vi "Arm Logic.vi"(8 "Button":bool=TRUE, 10 "Claw":bool=TRUE, 11 "Tote Count":dbl format="%#_13g") -> ()   [LabVIEW 2014]
uses:
  TypeDefs/SRE Enum.ctl
  Support Code/Robot Global Data.vi
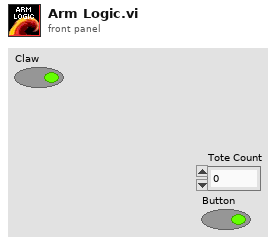
[diagram p1: front panel]
types:
  T1 = typedef "SRE Enum.ctl" = enum16{"Start", "Run", "End"}
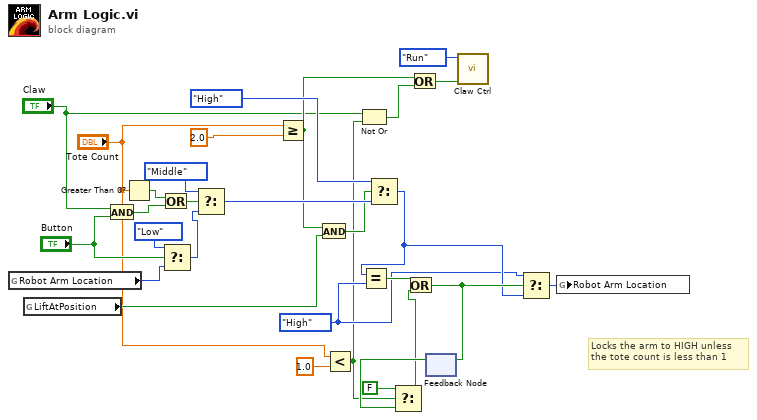
[diagram p0: block diagram]
diagram:
  w12 = enum16{"High", "Middle", "Low"}."High" ("y")
  # "Locks the arm to HIGH unless\nthe tote count is less than 1"
  n1 = global read "Robot Global Data.vi" "Robot Arm Location"() -> (w6:enum16{"High", "Middle", "Low"})
  n2 = global read "Robot Global Data.vi" "LiftAtPosition"() -> (w17:bool)
  n3 = And(x="Claw", y="Button") -> (x .and. y?=w23:bool)
  n4 = Greater Than 0?(x="Tote Count") -> (x > 0?=w24:bool)
  n5 = Or(x=w24, y=w23) -> (x .or. y?=w25:bool)
  n6 = Select(t=enum16{"High", "Middle", "Low"}."Low" ("Robot Arm Location"), s="Button", f=w6) -> (s? t:f=w21:enum16{"High", "Middle", "Low"})
  n7 = Select(t=enum16{"High", "Middle", "Low"}."Middle" ("Robot Arm Location"), s=w25, f=w21) -> (s? t:f=w26:enum16{"High", "Middle", "Low"})
  n8 = Greater Or Equal?(x="Tote Count", y=2.0) -> (x >= y?=w4:bool)
  n9 = And(x=w4, y=w17) -> (x .and. y?=w18:bool)
  n10 = Less?(x="Tote Count", y=1.0) -> (x < y?=w3:bool)
  n11 = Not Or(1:w3, 2:"Claw") -> (0:w1:bool)
  n12 = Select(t=enum16{"High", "Middle", "Low"}."High" ("Robot Arm Location"), s=w18, f=w26) -> (s? t:f=w14:enum16{"High", "Middle", "Low"})
  n13 = Equal?(x=w14, y=w12) -> (x = y?=w16:bool)
  n14 = Or(x=w4, y=w1) -> (x .or. y?=w22:bool)
  n15 = feedback #1() -> (w9:bool)  [unwired: 1 in]
  n16 = Select(t=FALSE, s=w3, f=w9) -> (s? t:f=w7:bool)
  n17 = Or(x=w16, y=w7) -> (x .or. y?=w15:bool)
  n18 = feedback-in #1(w15) -> ()
  n19 = call "Claw Ctrl.vi"("Open/Close"=w22, "Enum"=SRE_Enum."Run") -> ()  [unwired: 10 in]
  n20 = Select(t=w12, s=w15, f=w14) -> (s? t:f=w13:enum16{"High", "Middle", "Low"})
  n21 = global write "Robot Global Data.vi" "Robot Arm Location"(w13) -> ()
